vi "GetShortPathName.vi"(8 "Error In":errorcluster, 11 "Long Path In:":path=path "C:/My Documents/RealTime/Examples/Power Loss Recovery/Joes version/Splash Screen/Vibration Analysis.vi") -> (0 "Error Out":errorcluster, 3 "Short Path Out:":path, 5 "Operation Status:":string="Operation Succeeded")   [LabVIEW 2010]
doc: "This VI makes a call to the Windows Platform SDK function GetShortPathNameA that is part of the kernel32.dll. The GetShortPathNameA function converts long paths to the DOS short path format. A \"status\" output of 0 means the function failed."
uses:
  kernel32.dll
panel:
  out "Status:":u32
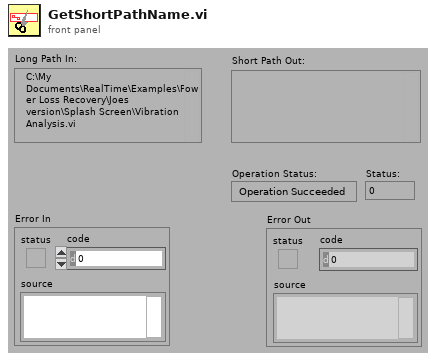
[diagram p1: front panel]
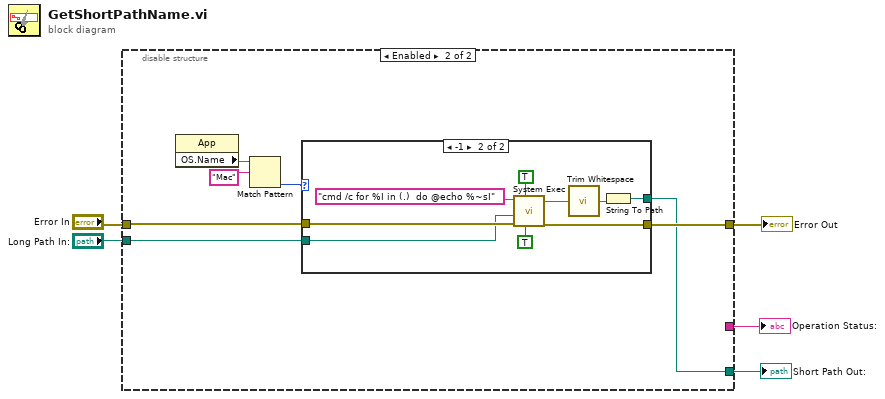
[diagram p0: block diagram]
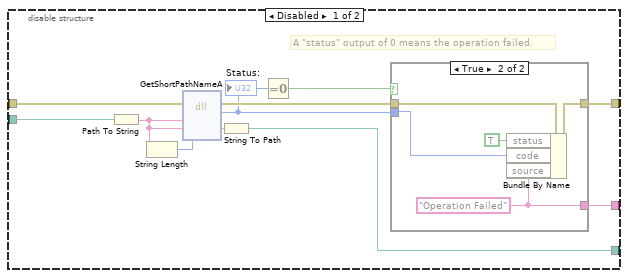
[diagram p2: hidden frame]
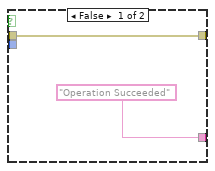
[diagram p3: hidden frame]
diagram:
  n1 = disable-structure shown="Enabled" {
    disable-tunnel: [w16 w28] -> w5
    disable-tunnel: [w11 _] -> w4
    disable-tunnel: "Long Path In:" -> [w10 w25]
    disable-tunnel: "Error In" -> [w9 w29]
    disable-tunnel: [w7 w30] -> w1
    frame Disabled {
      # "A \"status\" output of 0 means the operation failed."
      n2 = Path To String(path=w10) -> (string=w13:string)
      n3 = String Length(string=w13) -> (length=w15:i32)
      n4 = dll-call lib="kernel32.dll" fn="GetShortPathNameA"(error in=w9, "lpszLongPath"=w13, "lpszShortPath"=w13, "cchBuffer"=w15) -> (error out=w8:errorcluster, "status"=w6:u32, "lpszShortPath"=w14:string)  [unwired: 4 in, 1 out]
      "Status:" <- w6
      n5 = String To Path(string=w14) -> (path=w16:path)
      n6 = Equal To 0?(x=w6) -> (x = 0?=w12:bool)
      n7 = case shown="True" w12 {
        tunnel: ["Operation Succeeded" w20] -> w11
        tunnel: [w17 w22] -> w7
        tunnel: w8 -> [w17 w23]
        tunnel: w6 -> [_ w19]
        frame False {
        }
        frame True {
          w20 = "Operation Failed"
          n8 = Bundle By Name(cluster=w23, "status"=TRUE, "code"=w19, "source"=w20) -> (w22:errorcluster)
        }
      }
    }
    frame Enabled {
      n9 = property class="App"() -> ("OS.Name"=w27:string)  [unwired: 2 in, 2 out]
      n10 = Match Pattern(string=w27, regular expression="Mac") -> (offset past match=w24:i32)  [unwired: 1 in, 3 out]
      n11 = case shown="-1" w24 {
        tunnel: [w32 w41] -> w30
        tunnel: w29 -> [w32 w40]
        tunnel: [w31 w38] -> w28
        tunnel: w25 -> [w31 w33]
        frame Default {
        }
        frame -1 {
          n12 = call <vilib>:"System Exec.vi"("run minimized? (F)"=TRUE, "wait until completion? (T)"=TRUE, "error in (no error)"=w40, "working directory"=w33, "command line"="cmd /c for %I in (.)  do @echo %~sI") -> ("error out"=w41:errorcluster, "standard output"=w35:string)  [unwired: 3 in, 2 out]
          n13 = call <vilib>:"Trim Whitespace.vi"("string"=w35) -> ("trimmed string"=w34:string)  [unwired: 1 in]
          n14 = String To Path(string=w34) -> (path=w38:path)
        }
      }
    }
  }
  "Short Path Out:" <- w5
  "Operation Status:" <- w4
  "Error Out" <- w1
